vi "stage control.vi"(7 "Combo Box":string(combo), 8 "error in":errorcluster, 9 "speed":dbl=5.0, 10 "target":dbl, 11 "XPS Ref in":refnum<k24>) -> (0 "error out":errorcluster, 3 "XPS ref out":refnum<k24>)   [LabVIEW 2015]
uses:
  D:/labview program/whole brain TP_220607/sub vi/XPS-UNIFIED/LabVIEW VIs/LabVIEW Source Code/Dll/Newport.XPS.CommandInterface.dll
  XPS-UNIFIED/LabVIEW VIs/LabVIEW Source Code/Dll/Newport.XPS.CommandInterface.dll
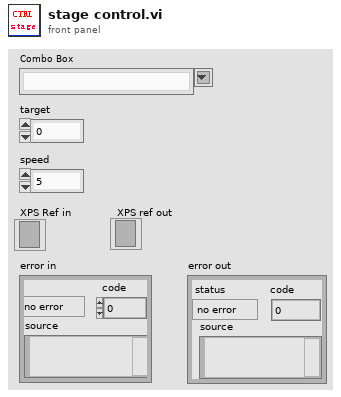
[diagram p1: front panel]
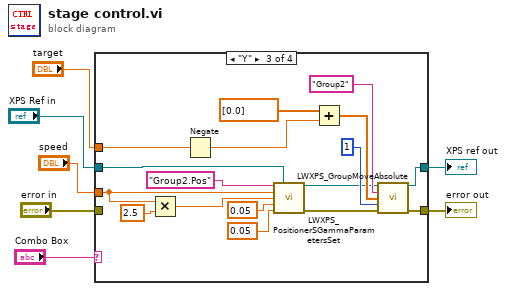
[diagram p0: block diagram]
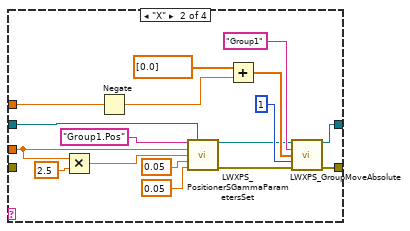
[diagram p3: hidden frame]
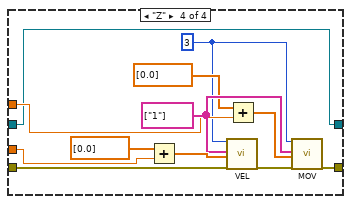
[diagram p4: hidden frame]
diagram:
  n1 = case shown="\"Y\"" "Combo Box" {
    tunnel: "speed" -> [_ w10 w29 w54]
    tunnel: "target" -> [_ w14 w27 w49]
    tunnel: "error in" -> [w9 _ _ w46]
    tunnel: [w9 w19 w36 w45] -> w3
    tunnel: "XPS Ref in" -> [w8 w18 w34 w44]
    tunnel: [w8 w17 w35 w44] -> w1
    frame "False", Default {
    }
    frame "X" {
      n2 = Multiply(x=w10, y=2.5) -> (x*y=w11:dbl)
      n3 = Negate(x=w14) -> (-x=w13:dbl)
      n4 = call "LWXPS_PositionerSGammaParametersSet.vi"("Positioner Name"="Group1.Pos", "CommandInterfaceXPS.XPS"=w18, "Motion velocity"=w10, "Motion acceleration"=w11, "Minimum jerk time"=0.05, "Maximum jerk time"=0.05) -> ("CommandInterfaceXPS.XPS"=w20:refnum<k24>, "LabVIEW error OUT"=w21:errorcluster)  [unwired: 6 in, 2 out]
      n5 = Add(x=dbl[] [0.0] ("Velocity values"), y=w13) -> (x+y=w23:dbl[])
      n6 = call "LWXPS_GroupMoveAbsolute.vi"("CommandInterfaceXPS.XPS"=w20, "Group Name"="Group1", "Target Position IN"=w23, "Number of Positioners"=1, "LabVIEW error IN"=w21) -> ("CommandInterfaceXPS.XPS"=w17:refnum<k24>, "LabVIEW error OUT"=w19:errorcluster)  [unwired: 6 in, 3 out]
    }
    frame "Y" {
      n7 = Multiply(x=w29, y=2.5) -> (x*y=w30:dbl)
      n8 = Negate(x=w27) -> (-x=w28:dbl)
      n9 = call "LWXPS_PositionerSGammaParametersSet.vi"("Positioner Name"="Group2.Pos", "CommandInterfaceXPS.XPS"=w34, "Motion velocity"=w29, "Motion acceleration"=w30, "Minimum jerk time"=0.05, "Maximum jerk time"=0.05) -> ("CommandInterfaceXPS.XPS"=w37:refnum<k24>, "LabVIEW error OUT"=w38:errorcluster)  [unwired: 6 in, 2 out]
      n10 = Add(x=dbl[] [0.0] ("Velocity values"), y=w28) -> (x+y=w40:dbl[])
      n11 = call "LWXPS_GroupMoveAbsolute.vi"("CommandInterfaceXPS.XPS"=w37, "Group Name"="Group2", "Target Position IN"=w40, "Number of Positioners"=1, "LabVIEW error IN"=w38) -> ("CommandInterfaceXPS.XPS"=w35:refnum<k24>, "LabVIEW error OUT"=w36:errorcluster)  [unwired: 6 in, 3 out]
    }
    frame "Z" {
      w48 = 3
      w51 = string[] ["1"] ("Axes to set")
      n12 = Add(x=dbl[] [0.0] ("Velocity values"), y=w54) -> (x+y=w55:dbl[])
      n13 = call "VEL.vi"("System no."=w48, "Axes to set"=w51, "Velocity values"=w55, "error in"=w46) -> ("error out"=w52:errorcluster)  [unwired: 2 in, 13 out]
      n14 = Add(x=dbl[] [0.0] ("Velocity values"), y=w49) -> (x+y=w47:dbl[])
      n15 = call "MOV.vi"("System no."=w48, "Axes to move"=w51, "Position values"=w47, "error in"=w52) -> ("error out"=w45:errorcluster)  [unwired: 1 in, 14 out]
    }
  }
  "error out" <- w3
  "XPS ref out" <- w1
